vi "Read Buffers.vi"(8 "error in (no error)":errorcluster, 11 "Data in":refnum<class "CV-Main.lvclass">) -> (0 "error out":errorcluster, 2 "Buffers":refnum<class "CV-Buffers.lvclass">, 3 "Data out":refnum<class "CV-Main.lvclass">)   [LabVIEW 2013, in "CameraVision.lvlib" / "CV-Main.lvclass"]
uses:
  CV-Main.lvclass
  Buffers/CV-Buffers.lvclass
  CV-Main.lvclass/CV-Main.ctl
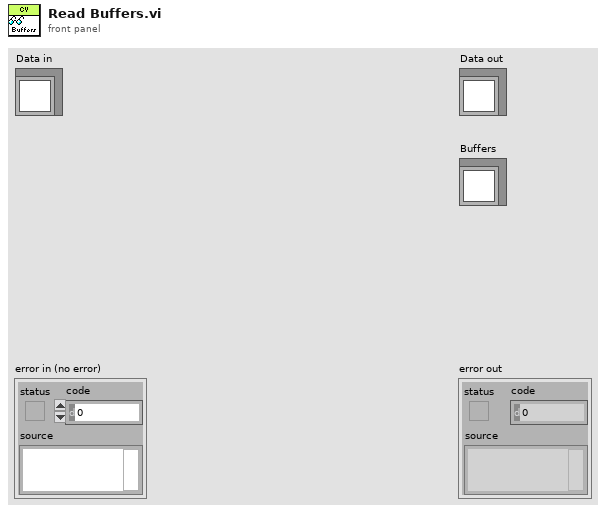
[diagram p1: front panel]
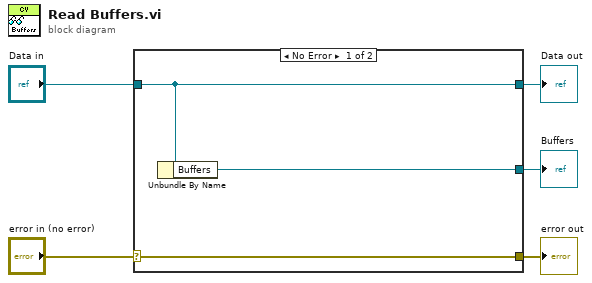
[diagram p0: block diagram]
diagram:
  n1 = case shown="No Error" "error in (no error)" {
    selector: "error in (no error)" -> [w8 w9]
    tunnel: [w8 w9] -> w4
    tunnel: [w7 w10] -> w2
    tunnel: "Data in" -> [w7 w10]
    tunnel: [w6 _] -> w1
    frame No Error {
      n2 = Unbundle By Name(w7) -> ("Buffers"=w6:refnum<class "CV-Buffers.lvclass">)
    }
    frame Error {
    }
  }
  "error out" <- w4
  "Data out" <- w2
  "Buffers" <- w1
